vi "Read files ALL(Sequence).vi"(11 "Path":path) -> (2 "Graph":dynamicdata(graph), 3 "Table":string[][](table))   [LabVIEW 2020, in "GPP.lvlib"]
uses:
  GPP.lvlib
panel:
  out "NUMBER":dbl[](array[numeric])
  out "N":dbl
  out "T":dbl
  out "C":dbl
  out "V":dbl
  out "TIME":dbl[](array[numeric])
  out "CURRENT":dbl[](array[numeric])
  out "VOLTAGE":dbl[](array[numeric])
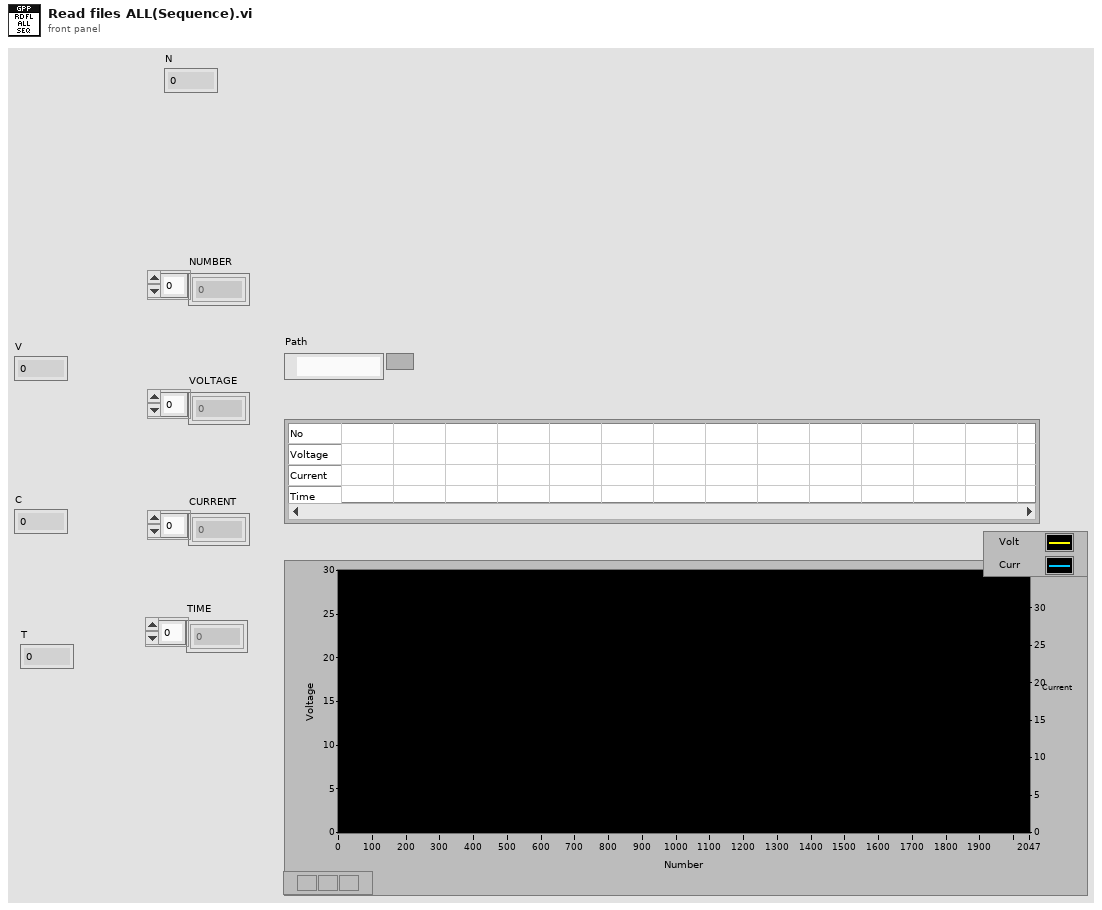
[diagram p1: front panel]
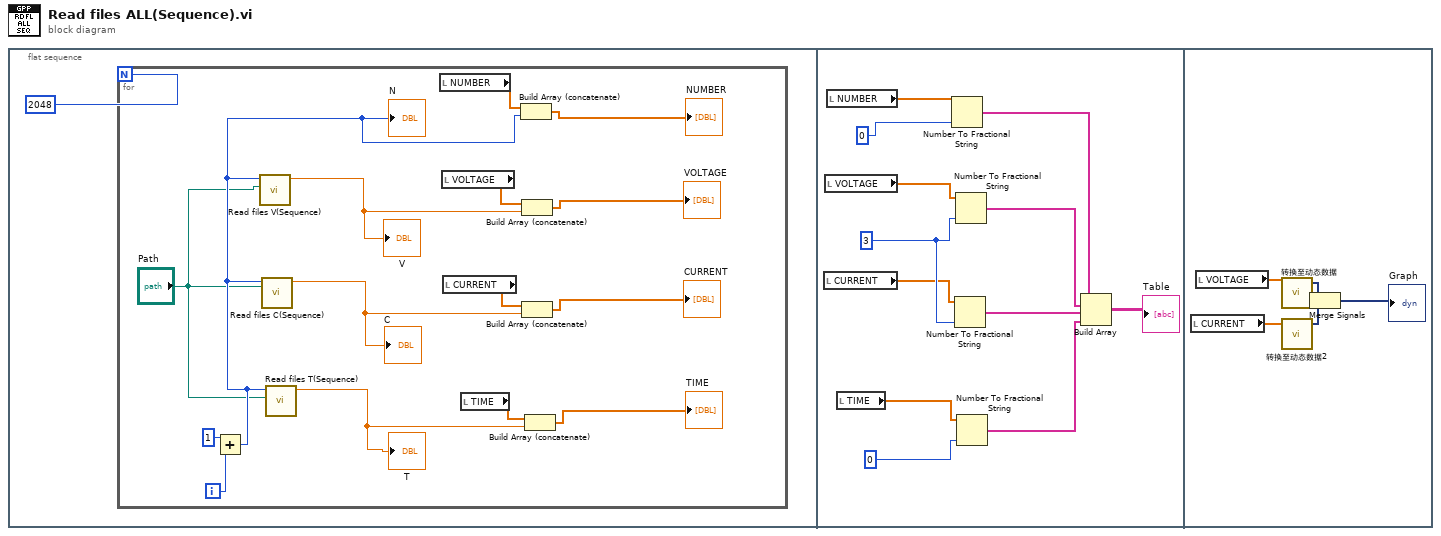
[diagram p0: block diagram]
diagram:
  n1 = flat-sequence {
    frame #0 {
      n2 = for {
        N: 2048 -> [_]
        i -> [w7]
        n3 = Add(x=1, y=w7) -> (x+y=w4:i32)
        "N" <- w4
        n4 = call "Read files V(Sequence).vi"("Path"="Path", "Number"=w4) -> ("Voltage"=w16:dbl)  [unwired: 9 in]
        "V" <- w16
        n5 = call "Read files C(Sequence).vi"("Path"="Path", "Number"=w4) -> ("Current"=w15:dbl)  [unwired: 9 in]
        "C" <- w15
        n6 = call "Read files T(Sequence).vi"("Path"="Path", "Number"=w4) -> ("Current"=w14:dbl)  [unwired: 9 in]
        "T" <- w14
        n7 = local read "NUMBER"() -> (w5:dbl[])
        n8 = local read "VOLTAGE"() -> (w13:dbl[])
        n9 = local read "CURRENT"() -> (w12:dbl[])
        n10 = local read "TIME"() -> (w11:dbl[])
        n11 = Build Array (concatenate)(w5, w4) -> (→"NUMBER":dbl[])
        n12 = Build Array (concatenate)(w13, w16) -> (→"VOLTAGE":dbl[])
        n13 = Build Array (concatenate)(w12, w15) -> (→"CURRENT":dbl[])
        n14 = Build Array (concatenate)(w11, w14) -> (→"TIME":dbl[])
      }
    }
    frame #1 {
      w23 = 3
      n15 = local read "CURRENT"() -> (w21:dbl[])
      n16 = local read "VOLTAGE"() -> (w20:dbl[])
      n17 = local read "NUMBER"() -> (w19:dbl[])
      n18 = local read "TIME"() -> (w22:dbl[])
      n19 = Number To Fractional String(number=w19, precision (6)=0) -> (F-format string=w17:string[])  [unwired: 2 in]
      n20 = Number To Fractional String(number=w21, precision (6)=w23) -> (F-format string=w26:string[])  [unwired: 2 in]
      n21 = Number To Fractional String(number=w20, precision (6)=w23) -> (F-format string=w25:string[])  [unwired: 2 in]
      n22 = Number To Fractional String(number=w22, precision (6)=0) -> (F-format string=w27:string[])  [unwired: 2 in]
      n23 = Build Array(w17, w25, w26, w27) -> (→"Table":string[][])
    }
    frame #2 {
      n24 = local read "CURRENT"() -> (w29:dbl[])
      n25 = local read "VOLTAGE"() -> (w30:dbl[])
      n26 = call "转换至动态数据"("Array"=w30) -> ("Dynamic Data Type"=w31:dynamicdata)  [unwired: 3 in]
      n27 = call "转换至动态数据2"("Array"=w29) -> ("Dynamic Data Type"=w32:dynamicdata)  [unwired: 3 in]
      n28 = Merge Signals(w31, w32) -> (→"Graph":dynamicdata)
    }
  }
